vi "Calibration-Frame4.vi"(9 "String":string, 10 "exists?":bool, 11 "Results file output":path) -> (1 "Output string":string, 2 "Boolean 2":bool, 3 "Boolean":bool)   [LabVIEW 2015]
uses:
  Anemometry Sub Vis/Globals/Calib_global.vi
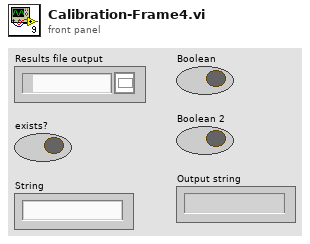
[diagram p1: front panel]
types:
  T1 = typedef "Cal_Inst_type.ctl" = enum16{"Propeller anemometer", "Pressure Transducer", "Hot wire", "Cross wire velocity", "Cross wire angle", "Generic Linear", "Generic Polynomial", "Generic BackPoly", "Fast FID", "Thermocouple", "Cold wire", "Pulsed Wire"}
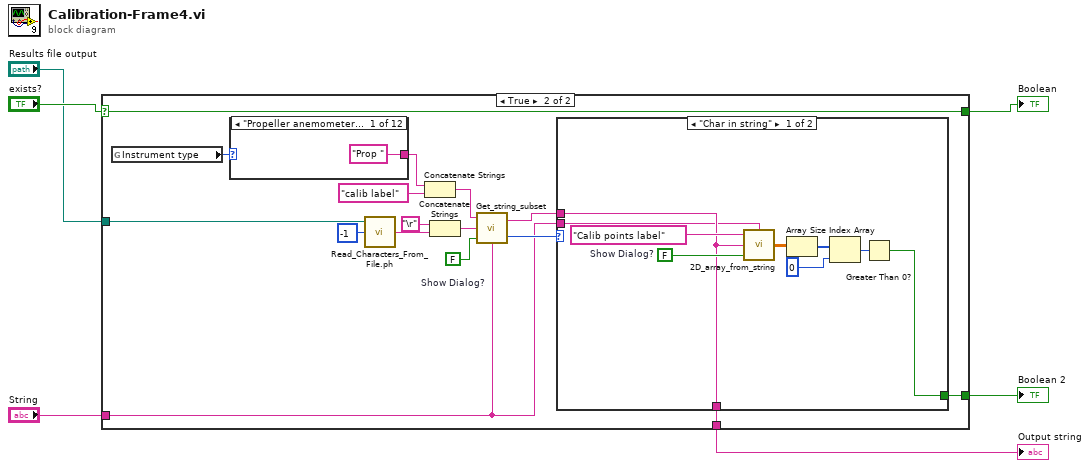
[diagram p0: block diagram]
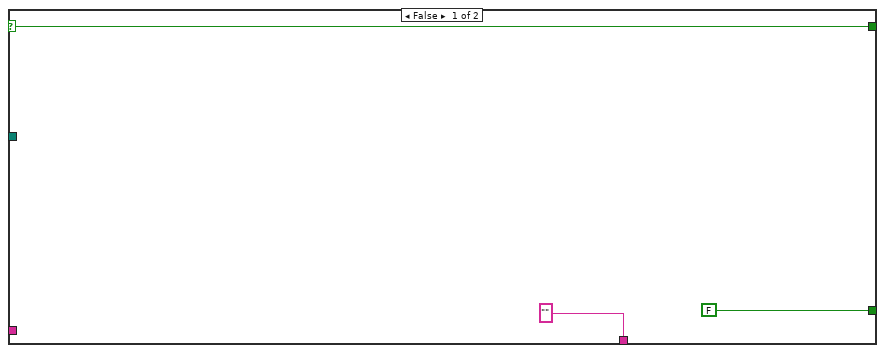
[diagram p2: hidden frame]
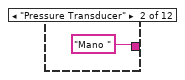
[diagram p3: hidden frame]
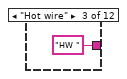
[diagram p4: hidden frame]
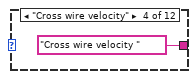
[diagram p5: hidden frame]
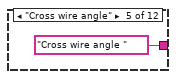
[diagram p6: hidden frame]
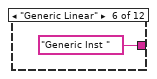
[diagram p7: hidden frame]
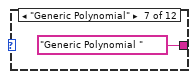
[diagram p8: hidden frame]
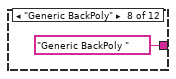
[diagram p9: hidden frame]
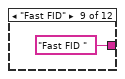
[diagram p10: hidden frame]
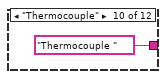
[diagram p11: hidden frame]
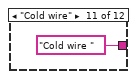
[diagram p12: hidden frame]
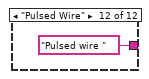
[diagram p13: hidden frame]
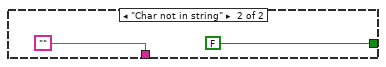
[diagram p14: hidden frame]
diagram:
  n1 = case shown="True" "exists?" {
    selector: "exists?" -> [w7 w10]
    tunnel: ["" ("Output string") w25] -> w1
    tunnel: [FALSE w24] -> w2
    tunnel: "Results file output" -> [_ w16]
    tunnel: "String" -> [_ w11]
    tunnel: [w7 w10] -> w6
    frame False {
    }
    frame True {
      w15 = FALSE  # Show Dialog?
      n2 = global read "Calib_global.vi" "Instrument type"() -> (w19:T1)
      n3 = case shown="\"Propeller anemometer\"" w19 {
        tunnel: ["Prop " "Mano " "HW " "Cross wire velocity " "Cross wire angle " "Generic Inst " "Generic Polynomial " "Generic BackPoly " "Fast FID " "Thermocouple " "Cold wire " "Pulsed wire "] -> w20
        frame "Propeller anemometer" {
        }
        frame "Pressure Transducer" {
        }
        frame "Hot wire" {
        }
        frame "Cross wire velocity" {
        }
        frame "Cross wire angle" {
        }
        frame "Generic Linear" {
        }
        frame "Generic Polynomial" {
        }
        frame "Generic BackPoly" {
        }
        frame "Fast FID" {
        }
        frame "Thermocouple" {
        }
        frame "Cold wire" {
        }
        frame "Pulsed Wire" {
        }
      }
      n4 = call "Read_Characters_From_File.ph.vi"("file path (dialog if empty)"=w16, "number of characters (all:-1)"=-1) -> ("character string"=w13:string)  [unwired: 7 out]
      n5 = Concatenate Strings(w20, "calib label") -> (w21:string)
      n6 = Concatenate Strings("\r", w13) -> (w12:string)
      n7 = call "Get_string_subset.vi"("String Name"=w11, "Show Dialog?"=w15, "String to split"=w12, "File Label"=w21) -> ("Status"=w18:enum16{"Char in string", "Char not in string"}, "Output string"=w17:string)
      n8 = case shown="\"Char in string\"" w18 {
        tunnel: w17 -> [w44 _]
        tunnel: [w44 ""] -> w25
        tunnel: [w39 FALSE] -> w24
        tunnel: w11 -> [w38 _]
        frame "Char in string" {
          w45 = FALSE  # Show Dialog?
          n9 = call "2D_array_from_string.vi"("String Name"=w38, "Show Dialog?"=w45, "Input string"=w44, "Array title"="Calib points label") -> ("2D data array"=w43:dbl[][])
          n10 = Array Size(array=w43) -> (size(s)=w42:i32[])
          n11 = Index Array(array=w42, index=0 ("Index")) -> (element=w40:i32)
          n12 = Greater Than 0?(x=w40) -> (x > 0?=w39:bool)
        }
        frame "Char not in string" {
        }
      }
    }
  }
  "Boolean" <- w6
  "Boolean 2" <- w2
  "Output string" <- w1
